vi "Okno_Czytaj_konwersje.vi"(7 "Path":path=path "D:/Marek/Dysk Google/Projekty LabVIEW/! Rudpol/Program/Konfiguracja/AI_konwersja.txt", 8 "error in":errorcluster, 10 "Wartosc In":T1={"X"="U", "[ ]"="V", "trans X"=1.0, "trans U"=1.0, "Z tabeli"=FALSE, "Opis"=""}) -> (0 "error out":errorcluster, 2 "Wartosc Out":T1={"X"="U", "[ ]"="V", "trans X"=1.0, "trans U"=1.0, "Z tabeli"=FALSE, "Opis"=""})   [LabVIEW 2014]
doc: "Otwiera okno wyboru i konfiguracji przetworników pomiarowych"
uses:
  Kontrolki/GUI/AI_wartosc.ctl
  <vilib>/Utility/config.llb/Read Key (String).vi
  <vilib>/Utility/config.llb/Read Key (Double).vi
  <vilib>/Utility/config.llb/Write Key (String).vi
  <vilib>/Utility/config.llb/Write Key (Double).vi
  <vilib>/Utility/config.llb/NI_LVConfig.lvlib
panel:
  out "Wybrano":T1={"X"="U", "[ ]"="V", "trans X"=1.0, "trans U"=1.0, "Z tabeli"=FALSE, "Opis"=""}
  in  "Uzupelnij":bool
  in  "Cancel Button":bool
  in  "OK Button":bool
  in  "Tabela":T1[](array[typedef])
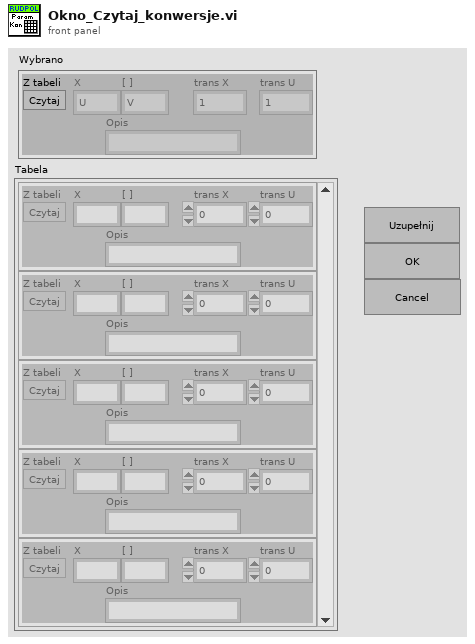
[diagram p1: front panel]
types:
  T1 = typedef "AI_wartosc.ctl" = cluster{"X":string, "[ ]":string, "trans X":dbl, "trans U":dbl, "Z tabeli":bool, "Opis":string}
  T2 = enum16{"open", "replace", "create", "open or create", "replace or create", "replace or create with confirmation"}
  T3 = typedef "NI_LVConfig.lvlib/Config Data RefNum.ctl" = refnum<k1>
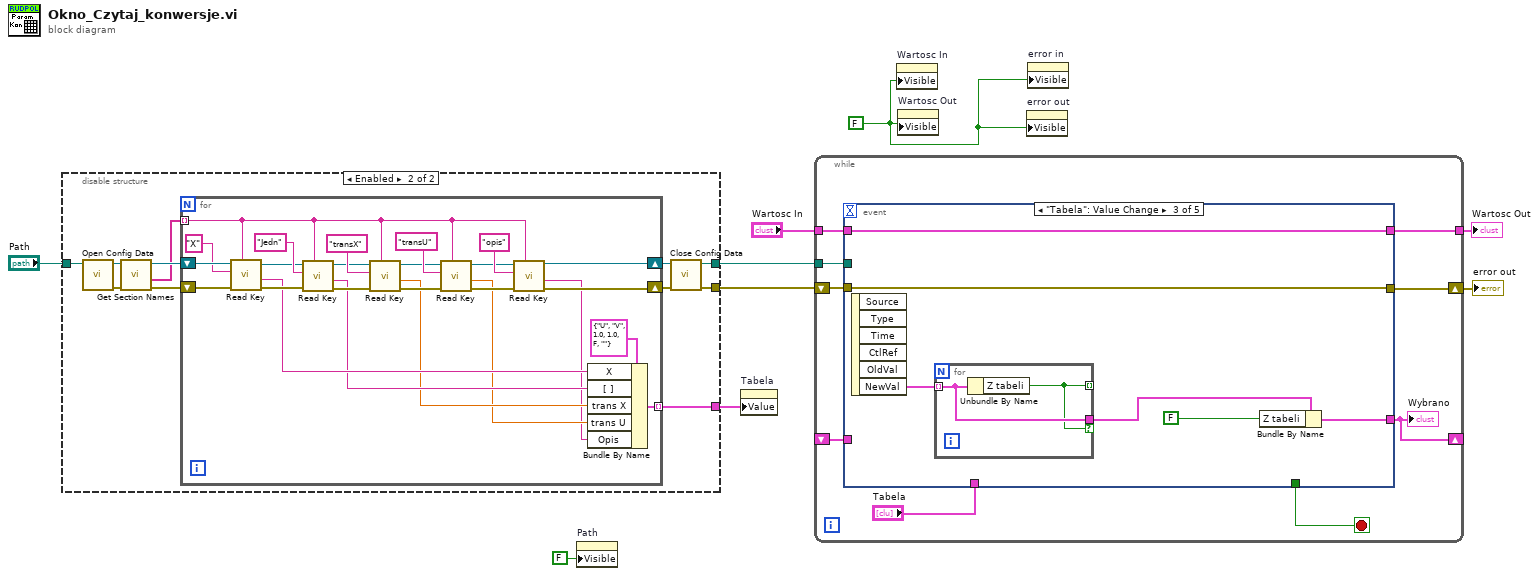
[diagram p0: block diagram]
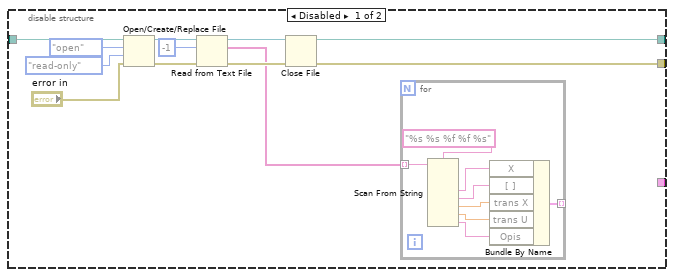
[diagram p2: hidden frame]
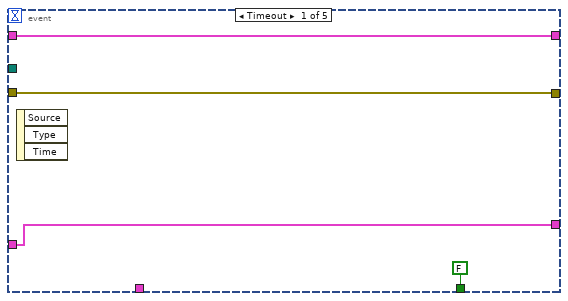
[diagram p3: hidden frame]
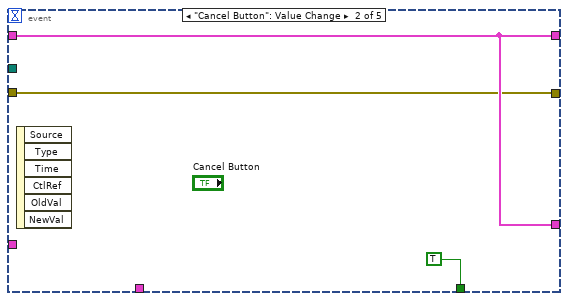
[diagram p4: hidden frame]
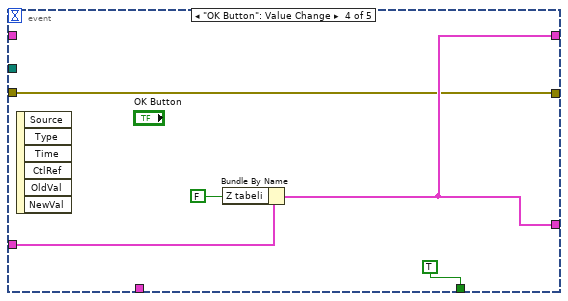
[diagram p5: hidden frame]
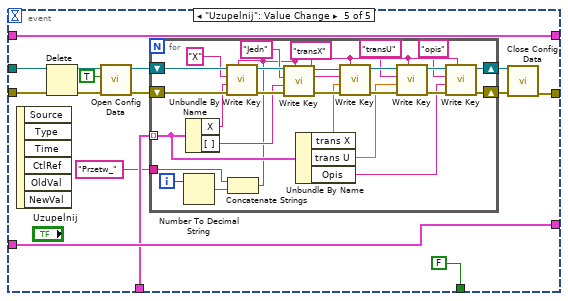
[diagram p6: hidden frame]
diagram:
  w3 = FALSE
  n1 = disable-structure shown="Enabled" {
    disable-tunnel: "Path" -> [w14 w38]
    disable-tunnel: [w13 w31] -> w8
    disable-tunnel: [w12 w33] -> w7
    disable-tunnel: [_ w34] -> w2
    frame Disabled {
      n2 = Open/Create/Replace File(file path (use dialog)=w14, error in="error in", operation (0:open)=T2."open", access (0:read/write)=enum16{"read/write", "read-only", "write-only"}."read-only") -> (refnum out=w18:refnum<file>, error out=w19:errorcluster)  [unwired: 2 in, 1 out]
      n3 = Read from Text File(file (use dialog)=w18, count=-1, error in=w19) -> (refnum out=w16:refnum<file>, text=w10:string[], error out=w17:errorcluster)  [unwired: 1 in, 1 out]
      n4 = Close File(refnum=w16, error in=w17) -> (path=w13:path, error out=w12:errorcluster)
      n5 = for {
        tunnel: [w24] -> _ mode=indexing
        tunnel: w10 -> [w22] mode=indexing
        n6 = Scan From String(format string="%s %s %f %f %s", input string=w22) -> (output 1=w28:string, output 2=w27:string, output 3=w26:dbl, output 4=w25:dbl, output 5=w23:string)  [unwired: 7 in, 3 out]
        n7 = Bundle By Name("X"=w28, "[ ]"=w27, "trans X"=w26, "trans U"=w25, "Opis"=w23) -> (w24:cluster{})  [unwired: 1 in]
      }
    }
    frame Enabled {
      n8 = call <vilib>:"Open Config Data.vi"("configuration file path"=w38) -> ("error out"=w40:errorcluster, "refnum"=w39:T3)  [unwired: 8 in, 1 out]
      n9 = call <vilib>:"Get Section Names.vi"("error in (no error)"=w40, "refnum"=w39) -> ("error out"=w37:errorcluster, "section names"=w35:string[], "refnum out"=w36:T3)  [unwired: 7 in]
      n10 = for {
        shift-right: [w59] -> w32
        shift-left: w37 -> [w65]
        tunnel: w35 -> [w58] mode=indexing
        tunnel: [w54] -> w34 mode=indexing
        shift-right: [w41] -> w30
        shift-left: w36 -> [w64]
        n11 = call-poly <vilib>:"Read Key.vi"("section"=w58, "error in (no error)"=w65, "key"="X", "refnum"=w64) -> ("error out"=w63:errorcluster, "value"=w56:string, "refnum out"=w42:T3)  [unwired: 4 in, 1 out]
        n12 = call-poly <vilib>:"Read Key.vi"("section"=w58, "error in (no error)"=w63, "key"="Jedn", "refnum"=w42) -> ("error out"=w62:errorcluster, "value"=w55:string, "refnum out"=w43:T3)  [unwired: 4 in, 1 out]
        n13 = call-poly <vilib>:"Read Key.vi"("section"=w58, "error in (no error)"=w62, "key"="transX", "refnum"=w43) -> ("error out"=w61:errorcluster, "value"=w52:dbl, "refnum out"=w44:T3)  [unwired: 4 in, 1 out]
        n14 = call-poly <vilib>:"Read Key.vi"("section"=w58, "error in (no error)"=w61, "key"="transU", "refnum"=w44) -> ("error out"=w60:errorcluster, "value"=w51:dbl, "refnum out"=w45:T3)  [unwired: 4 in, 1 out]
        n15 = call-poly <vilib>:"Read Key.vi"("section"=w58, "error in (no error)"=w60, "key"="opis", "refnum"=w45) -> ("error out"=w59:errorcluster, "value"=w50:string, "refnum out"=w41:T3)  [unwired: 4 in, 1 out]
        n16 = Bundle By Name(cluster=T1 {"X"="U", "[ ]"="V", "trans X"=1.0, "trans U"=1.0, "Z tabeli"=FALSE, "Opis"=""} ("Wartoœæ"), "X"=w56, "[ ]"=w55, "trans X"=w52, "trans U"=w51, "Opis"=w50) -> (w54:T1)
      }
      n17 = call <vilib>:"Close Config Data.vi"("error in (no error)"=w32, "refnum"=w30) -> ("error out"=w33:errorcluster, "file path"=w31:path)  [unwired: 8 in]
    }
  }
  n18 = property on="Path" class="Path"("Visible"=FALSE) -> ()  [unwired: 2 in, 2 out]
  n19 = property on="Tabela" class="Arr (strict)"("Value"=w2) -> ()  [unwired: 2 in, 2 out]
  n20 = while {
    tunnel: w8 -> [w74]
    shift-right: [w71] -> w4
    shift-left: w7 -> [w73]
    tunnel: [w69] -> w6
    tunnel: "Wartosc In" -> [w68]
    shift-right: [w67] -> _
    shift-left: _ -> [w66]
    stop <- w70 stop-if-true
    n21 = event shown="[2] \"Tabela\": Value Change" {
      selector: _ -> [_ _ _ _ _]
      dyn-events: _ -> [_ _ _ _ _]
      timeout: _ -> [_ _ _ _ _]
      tunnel: w74 -> [_ _ _ _ w105]
      tunnel: w73 -> [w77 w79 w85 w90 w104]
      tunnel: "Tabela" -> [_ _ _ _ w96]
      tunnel: [w77 w79 w85 w90 w106] -> w71
      tunnel: [FALSE TRUE _ TRUE FALSE] -> w70
      tunnel: [w75 w80 w86 w91 w107] -> w69
      tunnel: w68 -> [w75 w80 w86 _ w107]
      tunnel: [w76 w80 w83 w91 w108] -> w67
      tunnel: w66 -> [w76 _ _ w93 w108]
      event Timeout {
        n22 = event-data() -> ()  [unwired: 1 in, 3 out]
      }
      event "Cancel Button": Value Change {
        n23 = event-data() -> ()  [unwired: 1 in, 6 out]
      }
      event "Tabela": Value Change {
        n24 = event-data() -> ("NewVal"=w87:T1[])  [unwired: 1 in, 5 out]
        n25 = for {
          tunnel: w87 -> [w89] mode=indexing
          tunnel: [w88] -> _ mode=indexing
          tunnel: [w89] -> w84 if=w88
          n26 = Unbundle By Name(w89) -> ("Z tabeli"=w88:bool)
        }
        n27 = Bundle By Name(cluster=w84, "Z tabeli"=FALSE) -> (w83:T1)
      }
      event "OK Button": Value Change {
        n28 = event-data() -> ()  [unwired: 1 in, 6 out]
        n29 = Bundle By Name(cluster=w93, "Z tabeli"=FALSE) -> (w91:T1)
      }
      event "Uzupelnij": Value Change {
        n30 = event-data() -> ()  [unwired: 1 in, 6 out]
        n31 = Delete(path (use dialog)=w105, error in=w104) -> (deleted path=w102:path, error out=w103:errorcluster)  [unwired: 3 in, 1 out]
        n32 = call <vilib>:"Open Config Data.vi"("error in (no error)"=w103, "create file if necessary (T)"=TRUE, "configuration file path"=w102) -> ("error out"=w99:errorcluster, "refnum"=w100:T3)  [unwired: 6 in, 1 out]
        n33 = for {
          shift-right: [w125] -> w98
          shift-left: w99 -> [w135]
          shift-right: [w124] -> w97
          shift-left: w100 -> [w136]
          tunnel: w96 -> [w117] mode=indexing
          tunnel: "Przetw_" ("key") -> [w132]
          i -> [w134]
          n34 = Number To Decimal String(number=w134) -> (decimal integer string=w133:string)  [unwired: 1 in]
          n35 = Unbundle By Name(w117) -> ("X"=w129:string, "[ ]"=w127:string)
          n36 = Concatenate Strings(w132, w133) -> (w113:string)
          n37 = call-poly <vilib>:"Write Key.vi"("section"=w113, "error in (no error)"=w135, "value"=w129, "key"="X", "refnum"=w136) -> ("error out"=w131:errorcluster, "refnum out"=w130:T3)  [unwired: 4 in, 1 out]
          n38 = call-poly <vilib>:"Write Key.vi"("section"=w113, "error in (no error)"=w131, "value"=w127, "key"="Jedn", "refnum"=w130) -> ("error out"=w118:errorcluster, "refnum out"=w119:T3)  [unwired: 4 in, 1 out]
          n39 = Unbundle By Name(w117) -> ("trans X"=w116:dbl, "trans U"=w115:dbl, "Opis"=w114:string)
          n40 = call-poly <vilib>:"Write Key.vi"("section"=w113, "error in (no error)"=w118, "value"=w116, "key"="transX", "refnum"=w119) -> ("error out"=w120:errorcluster, "refnum out"=w121:T3)  [unwired: 4 in, 1 out]
          n41 = call-poly <vilib>:"Write Key.vi"("section"=w113, "error in (no error)"=w120, "value"=w115, "key"="transU", "refnum"=w121) -> ("error out"=w122:errorcluster, "refnum out"=w123:T3)  [unwired: 4 in, 1 out]
          n42 = call-poly <vilib>:"Write Key.vi"("section"=w113, "error in (no error)"=w122, "value"=w114, "key"="opis", "refnum"=w123) -> ("error out"=w125:errorcluster, "refnum out"=w124:T3)  [unwired: 4 in, 1 out]
        }
        n43 = call <vilib>:"Close Config Data.vi"("error in (no error)"=w98, "refnum"=w97) -> ("error out"=w106:errorcluster)  [unwired: 8 in, 1 out]
      }
    }
    "Wybrano" <- w67
  }
  "Wartosc Out" <- w6
  "error out" <- w4
  n44 = property on="Wartosc In" class="Clust (strict)"("Visible"=w3) -> ()  [unwired: 2 in, 2 out]
  n45 = property on="Wartosc Out" class="Clust (strict)"("Visible"=w3) -> ()  [unwired: 2 in, 2 out]
  n46 = property on="error out" class="Clust (strict)"("Visible"=w3) -> ()  [unwired: 2 in, 2 out]
  n47 = property on="error in" class="Clust (strict)"("Visible"=w3) -> ()  [unwired: 2 in, 2 out]
